vi "CRYScale Change.vi"(11 "Graph VI Ref":refnum<vi>) -> ()   [LabVIEW 2013]
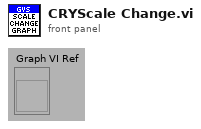
[diagram p1: front panel]
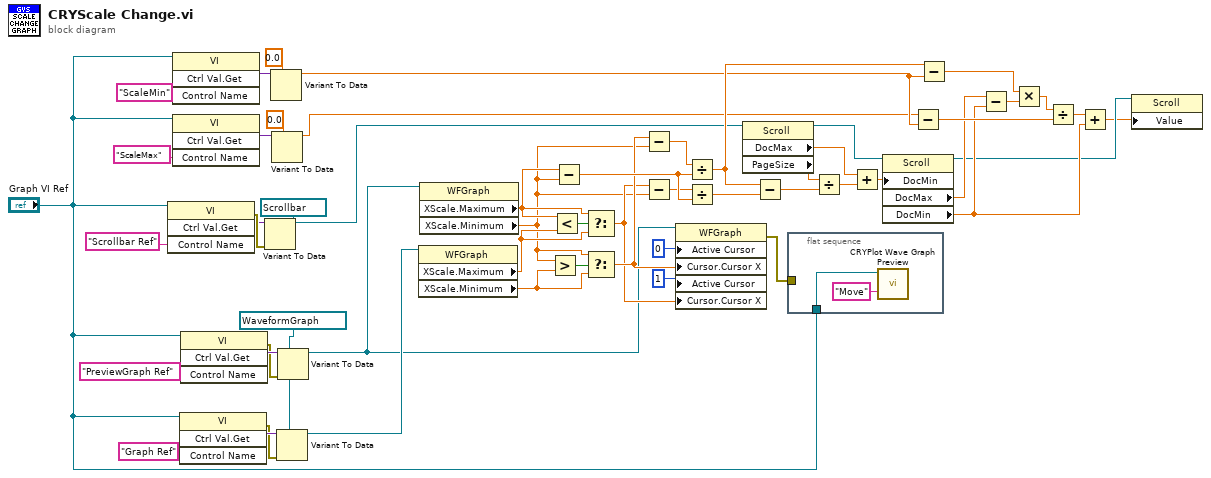
[diagram p0: block diagram]
diagram:
  w38 = refnum<vi> refnum ("Legend Ref")
  n1 = invoke class="VI" method="Ctrl Val.Get"(reference="Graph VI Ref", "Control Name"="Scrollbar Ref") -> (error out=w52:errorcluster, "Get Control Value Variant"=w51:variant)  [unwired: 2 in, 2 out]
  n2 = invoke class="VI" method="Ctrl Val.Get"(reference="Graph VI Ref", "Control Name"="ScaleMin") -> ("Get Control Value Variant"=w47:variant)  [unwired: 2 in, 3 out]
  n3 = invoke class="VI" method="Ctrl Val.Get"(reference="Graph VI Ref", "Control Name"="ScaleMax") -> ("Get Control Value Variant"=w50:variant)  [unwired: 2 in, 3 out]
  n4 = invoke class="VI" method="Ctrl Val.Get"(reference="Graph VI Ref", "Control Name"="Graph Ref") -> (error out=w39:errorcluster, "Get Control Value Variant"=w40:variant)  [unwired: 2 in, 2 out]
  n5 = invoke class="VI" method="Ctrl Val.Get"(reference="Graph VI Ref", "Control Name"="PreviewGraph Ref") -> (error out=w43:errorcluster, "Get Control Value Variant"=w44:variant)  [unwired: 2 in, 2 out]
  n6 = Variant To Data(error in=w52, type=refnum<vi> refnum ("Legend Ref"), Variant=w51) -> (data=w7:refnum<vi>)  [unwired: 1 out]
  n7 = Variant To Data(type=0.0 ("X Scale.Range:Maximum"), Variant=w47) -> (data=w9:dbl)  [unwired: 1 in, 1 out]
  n8 = Variant To Data(type=0.0 ("X Scale.Range:Maximum"), Variant=w50) -> (data=w8:dbl)  [unwired: 1 in, 1 out]
  n9 = Variant To Data(error in=w39, type=w38, Variant=w40) -> (data=w6:refnum<vi>)  [unwired: 1 out]
  n10 = Variant To Data(error in=w43, type=w38, Variant=w44) -> (data=w1:refnum<vi>)  [unwired: 1 out]
  n11 = property on="Property Node" class="WFGraph"(reference=w6) -> ("XScale.Maximum"=w35:dbl, "XScale.Minimum"=w36:dbl)  [unwired: 1 in, 2 out]
  n12 = property on="Property Node" class="WFGraph"(reference=w1) -> ("XScale.Maximum"=w22:dbl, "XScale.Minimum"=w16:dbl)  [unwired: 1 in, 2 out]
  n13 = Greater?(x=w16, y=w36) -> (0:w37:bool)
  n14 = Less?(x=w22, y=w35) -> (x < y?=w34:bool)
  n15 = Subtract(x=w22, y=w16) -> (x-y=w21:dbl)
  n16 = Select(t=w22, s=w34, f=w35) -> (s? t:f=w17:dbl)
  n17 = Select(t=w16, s=w37, f=w36) -> (s? t:f=w18:dbl)
  n18 = Subtract(x=w18, y=w16) -> (x-y=w15:dbl)
  n19 = Subtract(x=w17, y=w16) -> (x-y=w14:dbl)
  n20 = property on="Property Node" class="WFGraph"(reference=w1, "Active Cursor"=u32 0, "Cursor.Cursor X"=w18, "Active Cursor"=u32 1, "Cursor.Cursor X"=w17) -> (error out=w33:errorcluster)  [unwired: 1 in, 1 out]
  n21 = Divide(x=w15, y=w21) -> (x/y=w19:dbl)
  n22 = Divide(x=w14, y=w21) -> (x/y=w20:dbl)
  n23 = property on="Property Node" class="Scroll"(reference=w7) -> (reference out=w5:refnum<vi>, "DocMax"=w26:dbl, "PageSize"=w10:dbl)  [unwired: 1 in, 1 out]
  n24 = Subtract(x=w19, y=w20) -> (x-y=w24:dbl)
  n25 = flat-sequence {
    tunnel: w33 -> [_]
    tunnel: "Graph VI Ref" -> [w55]
    frame #0 {
      n26 = call "CRYPlot Wave Graph Preview.vi"("sOption"="Move", "Graph VI Ref"=w55) -> ()  [unwired: 10 in]
    }
  }
  n27 = Divide(x=w10, y=w24) -> (x/y=w23:dbl)
  n28 = Add(x=w26, y=w23) -> (x+y=w25:dbl)
  n29 = property on="Property Node" class="Scroll"(reference=w5, "DocMin"=w25) -> (reference out=w4:refnum<vi>, "DocMax"=w12:dbl, "DocMin"=w11:dbl)  [unwired: 1 in, 1 out]
  n30 = Subtract(x=w8, y=w9) -> (x-y=w13:dbl)
  n31 = Subtract(x=w19, y=w9) -> (x-y=w27:dbl)
  n32 = Subtract(x=w12, y=w11) -> (x-y=w28:dbl)
  n33 = Multiply(x=w27, y=w28) -> (x*y=w29:dbl)
  n34 = Divide(x=w29, y=w13) -> (x/y=w30:dbl)
  n35 = Add(x=w30, y=w11) -> (x+y=w3:dbl)
  n36 = property on="Property Node" class="Scroll"(reference=w4, "Value"=w3) -> ()  [unwired: 1 in, 2 out]
